vi "VisionDashReadSlow.vi"(8 "error in (no error)":errorcluster) -> (0 "error out":errorcluster)   [LabVIEW 2023]
doc: "Vision Network\n\nInput\n --Error in \n\nOutput\n --Error out"
uses:
  <vilib>/Rock Robotics/WPI/ThirdParty/JAS_Junk/TrajLib/Trajectory_Library.lvlib
  <vilib>/Rock Robotics/Network Tables/NT Read Number.vi
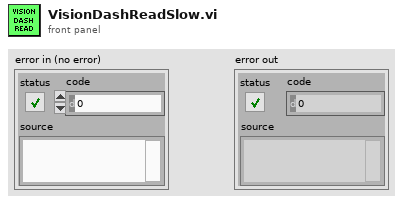
[diagram p1: front panel]
types:
  T1 = typedef "Trajectory_Library.lvlib/POSE2D.ctl" = cluster{"TRANSLATION":T2, "ROTATION":T3}
  T2 = typedef "Trajectory_Library.lvlib/TRANSLATION2D.ctl" = cluster{"X":dbl, "Y":dbl}
  T3 = typedef "Trajectory_Library.lvlib/ROTATION2D.ctl" = cluster{"VALUE":dbl, "COS":dbl, "SIN":dbl}
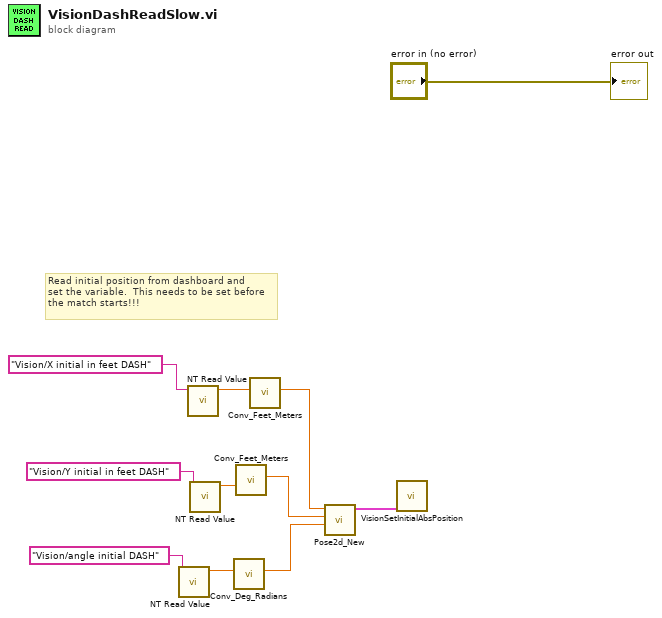
[diagram p0: block diagram]
diagram:
  # "Read initial position from dashboard and\nset the variable.  This needs to be set before\nthe match starts!!!"
  n1 = call-poly <vilib>:"NT Read Value.vi"("name"="Vision/angle initial DASH") -> ("value"=w5:dbl)  [unwired: 8 in, 2 out]
  n2 = call-poly <vilib>:"NT Read Value.vi"("name"="Vision/X initial in feet DASH") -> ("value"=w8:dbl)  [unwired: 8 in, 2 out]
  n3 = call-poly <vilib>:"NT Read Value.vi"("name"="Vision/Y initial in feet DASH") -> ("value"=w7:dbl)  [unwired: 8 in, 2 out]
  n4 = call <vilib>:"Conv_Deg_Radians.vi"("Degress"=w5) -> ("Radians"=w4:dbl)  [unwired: 10 in]
  n5 = call <vilib>:"Conv_Feet_Meters.vi"("Feet"=w7) -> ("Meters"=w6:dbl)  [unwired: 10 in]
  n6 = call <vilib>:"Conv_Feet_Meters.vi"("Feet"=w8) -> ("Meters"=w9:dbl)  [unwired: 10 in]
  n7 = call <vilib>:"Pose2d_New.vi"("Heading"=w4, "Y"=w6, "X"=w9) -> ("out POSe"=w10:T1)  [unwired: 8 in]
  n8 = call "VisionSetInitialAbsPosition.vi"("InitialPose"=w10) -> ()  [unwired: 11 in]
  "error out" <- "error in (no error)"
